vi "Prep Data for Graph.vi"(1 "Data":sgl[][](array[numeric]), 7 "Graph Ch Refs":refnum<vi>[](array[refnum]), 11 "Pretrigger Size":i32, 12 "Buffer Size":u32) -> (3 "Elements Deleted":dbl, 8 "Current Size":dbl, 14 "Data Out":sgl[][](array[numeric]))   [LabVIEW 2023]
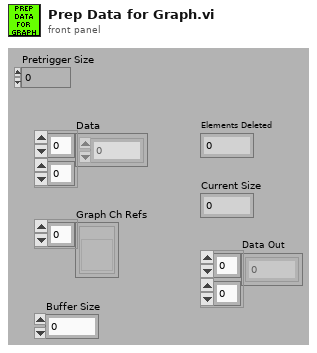
[diagram p1: front panel]
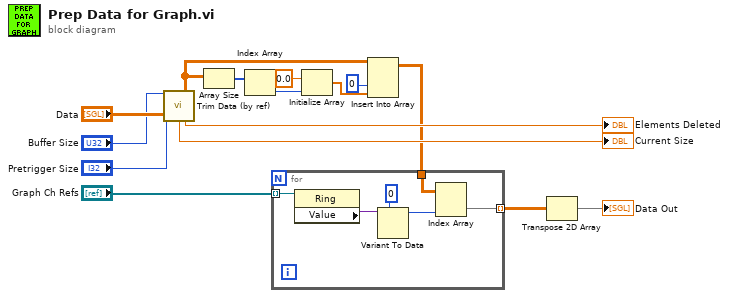
[diagram p0: block diagram]
diagram:
  n1 = call "Trim Data (by ref).vi"("length"="Buffer Size", "Pretrigger Size"="Pretrigger Size", "Array"="Data") -> ("Data Out"=w13:sgl[][], "Current Size"=→"Current Size":dbl, "Elements Deleted"=→"Elements Deleted":dbl)  [unwired: 10 in]
  n2 = Array Size(array=w13) -> (size(s)=w6:i32[])
  n3 = Index Array(array=w6) -> (element=w10:i32)  [unwired: 1 in]
  n4 = Initialize Array(sgl 0.0 ("element"), w10) -> (w4:sgl[])
  n5 = Insert Into Array(array=w13, index (col)=0 ("index (row)"), new element=w4) -> (w9:sgl[][])  [unwired: 1 in]
  n6 = for {
    tunnel: "Graph Ch Refs" -> [w21] mode=indexing
    tunnel: w9 -> [w20]
    tunnel: [w16] -> w8 mode=indexing
    n7 = property class="Ring"(reference=w21) -> ("Value"=w18:variant)  [unwired: 1 in, 2 out]
    n8 = Variant To Data(type=u16 0, Variant=w18) -> (data=w17:u16)  [unwired: 1 in, 1 out]
    n9 = Index Array(array=w20, index (col)=w17) -> (element=w16:sgl[])  [unwired: 1 in]
  }
  n10 = Transpose 2D Array(2D array=w8) -> (transposed array=→"Data Out":sgl[][])
